vi "TeddingtonClient.vi"() -> (0 "Time Of Value (s)":dbl format="%#.1f", 1 "Error":bool, 2 "Sea level Pressure String/mBar":dbl)   [LabVIEW 2011]
panel:
  out "Time Stamp GMT":timestamp
  out "data out":string
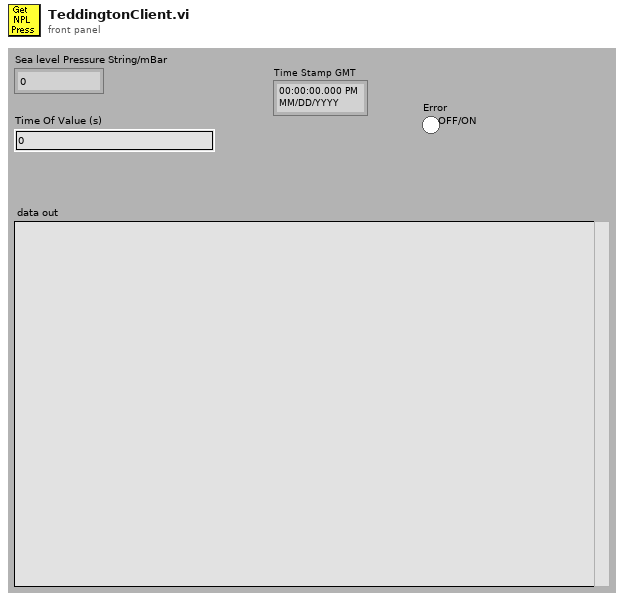
[diagram p1: front panel]
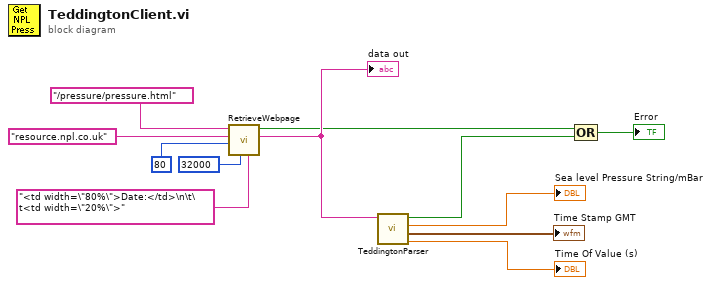
[diagram p0: block diagram]
diagram:
  n1 = call "RetrieveWebpage.vi"("lastStringRequired"="<td width=\"80%\">Date:</td>\n\t\t<td width=\"20%\">", "minimumBytesToRead"=32000, "port"=u16 80 ("remote port"), "server"="resource.npl.co.uk" ("address"), "pageURL"="/pressure/pressure.html" ("data in")) -> ("webpageOut"=w7:string, "TCPerror"=w1:bool)  [unwired: 5 in]
  "data out" <- w7
  n2 = call "TeddingtonParser.vi"("webpage"=w7) -> ("timeOfValue"=→"Time Of Value (s)":dbl, "Time Stamp GMT"=→"Time Stamp GMT":timestamp, "SeaLevelPressure"=→"Sea level Pressure String/mBar":dbl, "NotFound"=w10:bool)  [unwired: 7 in]
  n3 = Compound Arithmetic op=OR(w1, w10) -> (→"Error":bool)
